vi "ReadState.vi"(8 "Error In":errorcluster, 9 "Timeout":i32=-1, 11 "Queue In":refnum<queue>) -> (0 "Error Out":errorcluster, 1 "Data":variant, 2 "State":string, 3 "Queue Out":refnum<queue>)   [LabVIEW 2014]
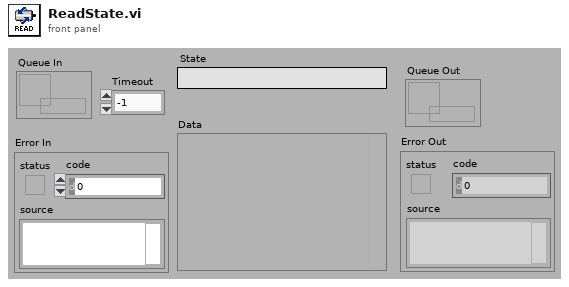
[diagram p1: front panel]
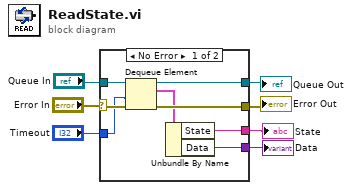
[diagram p0: block diagram]
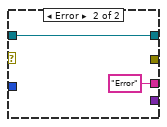
[diagram p2: hidden frame]
diagram:
  n1 = case shown="No Error" "Error In" {
    selector: "Error In" -> [w15 _]
    tunnel: [w14 _] -> w6
    tunnel: [w13 w17] -> w5
    tunnel: "Queue In" -> [w12 w17]
    tunnel: [w10 "Error" ("State")] -> w3
    tunnel: [w9 _] -> w2
    tunnel: "Timeout" -> [w8 _]
    frame No Error {
      n2 = Dequeue Element(queue=w12, timeout in ms (-1)=w8, error in (no error)=w15) -> (queue out=w13:refnum<queue>, element=w11:cluster{"State":string, "Data":variant}, error out=w14:errorcluster)  [unwired: 1 out]
      n3 = Unbundle By Name(w11) -> ("State"=w10:string, "Data"=w9:variant)
    }
    frame Error {
    }
  }
  "Data" <- w2
  "State" <- w3
  "Queue Out" <- w5
  "Error Out" <- w6
